vi "Change Tag.vi"(6 "Variant":variant, 8 "error in (no error)":errorcluster, 9 "old values":string[][](array[string]), 10 "object ref in":T1, 11 "Cluster":T2) -> (0 "error out":errorcluster)   [LabVIEW 2013, in "current tag file io module editor node.lvclass"]
uses:
  current tag file io module editor node.lvclass
  <vilib>/NI/DCAF Table API/Table Manager/Cell Change.ctl
  <vilib>/NI/DCAF Table API/Table Manager/object ref.ctl
  <vilib>/NI/Tag Bus Data Framework/Configuration Editor/Classes/Engine Parent/Engine Parent Editor Node.lvclass
  <vilib>/NI/Tag Bus Data Framework/Configuration Editor/Classes/Module editor node/module editor node.lvclass
  <vilib>/NI/Tag Bus Module Framework/channel/TBM channel.lvclass
  <vilib>/NI/Tag Bus/tag/tag descriptor.lvclass/tag descriptor.ctl
  module/configuration/current tag file io module configuration.lvclass
  module/configuration/current tag file io module configuration.lvclass/current tag file io module configuration.ctl
  <vilib>/NI/Tag Bus/tag/tag descriptor.lvclass
  <vilib>/NI/DCAF Table API/Table Manager.lvlib
  <vilib>/NI/DCAF Table API/Table Manager/Table Manager.lvclass
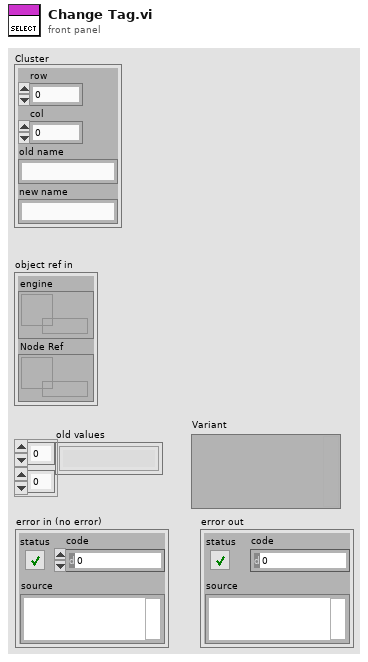
[diagram p1: front panel]
types:
  T1 = typedef "Table Manager.lvlib/Table Manager.lvclass/object ref.ctl" = cluster{"engine":refnum<data-value>, "Node Ref":refnum<data-value>}
  T2 = typedef "Table Manager.lvlib/Cell Change.ctl" = cluster{"row":i32, "col":i32, "old name":string, "new name":string}
  T3 = typedef "current tag file io module configuration.lvclass/tag configuration.ctl" = cluster{"name":string, "data type":T4, "channel":refnum<class "TBM channel.lvclass">}
  T4 = typedef "tag bus.lvlib/tag descriptor.lvclass/Data Type.ctl" = enum16{"Double", "Single", "I64", "I32", "I16", "I8", "U64", "U32", "U16", "U8", "Boolean", "String", "Array of Double", "Array of Single", "Array of I64", "Array of I32", "Array of I16", "Array of I8", "Array of U64", "Array of U32", "Array of U16", "Array of U8", "Array of Boolean", "Array of String"}
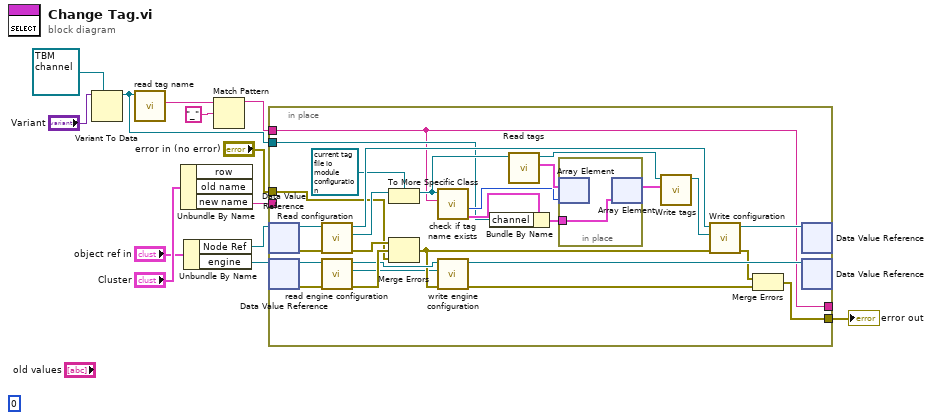
[diagram p0: block diagram]
diagram:
  (unwired) 0 ("disabled index (col)")
  n1 = Variant To Data(type=refnum<class "TBM channel.lvclass"> refnum ("output"), Variant="Variant") -> (data=w2:refnum<class "TBM channel.lvclass">)  [unwired: 1 in, 1 out]
  n2 = call <vilib>:"read tag name.vi"("system tag in"=w2) -> ("name"=w4:string)  [unwired: 8 in, 2 out]
  n3 = Unbundle By Name("Cluster") -> ("new name"=w7:string)  [unwired: 2 out]
  n4 = Unbundle By Name("object ref in") -> ("Node Ref"=w9:refnum<data-value>, "engine"=w8:refnum<data-value>)
  n5 = Match Pattern(string=w4, regular expression="_") -> (before substring=w1:string)  [unwired: 1 in, 3 out]
  n6 = in-place {
    in-place-border: [w33] -> w13
    in-place-border: "error in (no error)" -> [w25]
    in-place-border: [w14] -> _
    in-place-border: w7 -> [_]
    in-place-border: w2 -> [w15]
    in-place-border: w1 -> [w14]
    n7 = in-place-dvr #1(w9) -> (w30:refnum<class "module editor node.lvclass">, w32:errorcluster)
    n8 = in-place-dvr #2(w8) -> (w40:refnum<class "Engine Parent Editor Node.lvclass">, w41:errorcluster)
    n9 = call-dynamic "Read configuration.vi"("error in"=w32, "NISE_CEF_serializable node in"=w30) -> ("error out"=w31:errorcluster, "configuration"=w28:refnum<class "NISE_CEF_serializable configuration.lvclass">, "NISE_CEF_serializable node out"=w29:refnum<class "module editor node.lvclass">)  [unwired: 7 in]
    n10 = call <vilib>:"read engine configuration.vi"("error in"=w41, "Engine Parent Editor Node in"=w40) -> ("error out"=w37:errorcluster, "engine configuration"=w16:refnum<class "engine configuration.lvclass">, "Engine Parent Editor Node out"=w36:refnum<class "Engine Parent Editor Node.lvclass">)  [unwired: 7 in]
    n11 = To More Specific Class(target class=refnum<class "current tag file io module configuration.lvclass"> refnum ("tag select module configuration"), reference=w28) -> (specific class reference=w24:refnum<class "current tag file io module configuration.lvclass">)  [unwired: 1 in, 1 out]
    n12 = Merge Errors(w31, w37, w25) -> (w27:errorcluster)
    n13 = call "check if tag name exists.vi"("name to locate"=w14, "configuration in"=w24) -> ("tag config"=w19:T3, "index"=w20:i32)  [unwired: 6 in, 2 out]
    n14 = call <vilib>:"write engine configuration.vi"("error in"=w27, "engine configuration"=w16, "Engine Parent Editor Node in"=w36) -> ("error out"=w35:errorcluster, "Engine Parent Editor Node out"=w39:refnum<class "Engine Parent Editor Node.lvclass">)  [unwired: 7 in]
    n15 = Bundle By Name(cluster=w19, "channel"=w15) -> (w18:T3)
    n16 = call "Read tags.vi"("current tag file io module configuration in"=w24) -> ("tags"=w23:T3[], "current tag file io module configuration out"=w21:refnum<class "current tag file io module configuration.lvclass">)  [unwired: 8 in, 1 out]
    n17 = in-place {
      in-place-border: w18 -> [w42]
      n18 = in-place-array #3(w23, w20) -> ()  [unwired: 1 out]
      n19 = in-place-array #3(w42) -> (w22:T3[])  [unwired: 1 out]
    }
    n20 = call "Write tags.vi"("tags"=w22, "current tag file io module configuration in"=w21) -> ("current tag file io module configuration out"=w17:refnum<class "current tag file io module configuration.lvclass">)  [unwired: 8 in, 1 out]
    n21 = call-dynamic "Write configuration.vi"("error in"=w27, "configuration"=w17, "NISE_CEF_serializable node in"=w29) -> ("error out"=w34:errorcluster, "NISE_CEF_serializable node out"=w38:refnum<class "module editor node.lvclass">)  [unwired: 7 in]
    n22 = Merge Errors(w34, w35) -> (w33:errorcluster)
    n23 = in-place-dvr #1(w38) -> ()  [unwired: 2 out]
    n24 = in-place-dvr #2(w39) -> ()  [unwired: 2 out]
  }
  "error out" <- w13
